vi "USB Get Device Info.vi"(10 "pFunctionStr":string, 11 "DevIndex":i32) -> (1 "function return":bool, 2 "pFunctionStr out":string, 3 "pDevInfo":T1)   [LabVIEW 2010, in "usb_device.lvlib"]
doc: "bool WINAPI USB_GetDeviceInfo(int DevIndex,PDEVICE_INFO pDevInfo,char *pFunctionStr);"
uses:
  usb_device.lvlib
  USB2XXX.dll
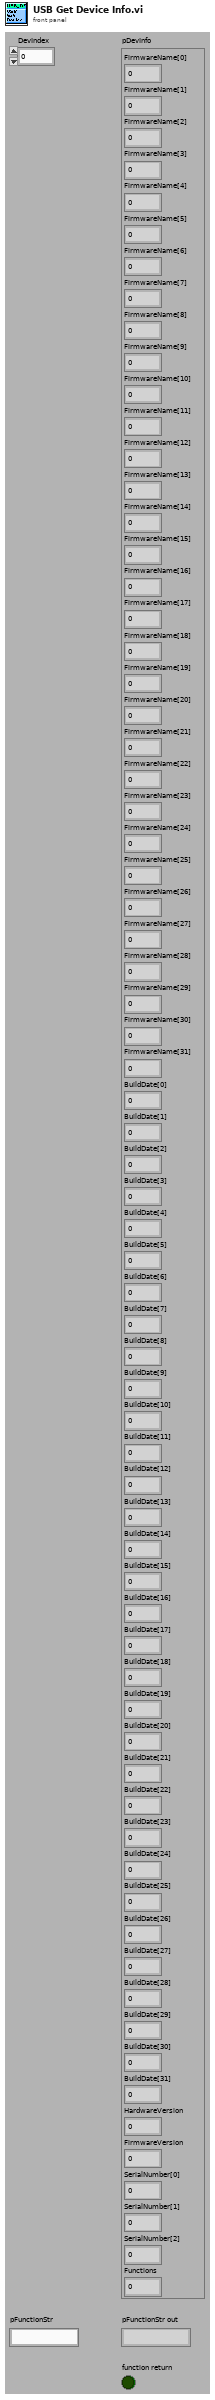
[diagram p1: front panel]
types:
  T1 = cluster{"FirmwareName[0]":i8, "FirmwareName[1]":i8, "FirmwareName[2]":i8, "FirmwareName[3]":i8, "FirmwareName[4]":i8, "FirmwareName[5]":i8, "FirmwareName[6]":i8, "FirmwareName[7]":i8, "FirmwareName[8]":i8, "FirmwareName[9]":i8, "FirmwareName[10]":i8, "FirmwareName[11]":i8, "FirmwareName[12]":i8, "FirmwareName[13]":i8, "FirmwareName[14]":i8, "FirmwareName[15]":i8, "FirmwareName[16]":i8, "FirmwareName[17]":i8, "FirmwareName[18]":i8, "FirmwareName[19]":i8, "FirmwareName[20]":i8, "FirmwareName[21]":i8, "FirmwareName[22]":i8, "FirmwareName[23]":i8, "FirmwareName[24]":i8, "FirmwareName[25]":i8, "FirmwareName[26]":i8, "FirmwareName[27]":i8, "FirmwareName[28]":i8, "FirmwareName[29]":i8, "FirmwareName[30]":i8, "FirmwareName[31]":i8, "BuildDate[0]":i8, "BuildDate[1]":i8, "BuildDate[2]":i8, "BuildDate[3]":i8, "BuildDate[4]":i8, "BuildDate[5]":i8, "BuildDate[6]":i8, "BuildDate[7]":i8, "BuildDate[8]":i8, "BuildDate[9]":i8, "BuildDate[10]":i8, "BuildDate[11]":i8, "BuildDate[12]":i8, "BuildDate[13]":i8, "BuildDate[14]":i8, "BuildDate[15]":i8, "BuildDate[16]":i8, "BuildDate[17]":i8, "BuildDate[18]":i8, "BuildDate[19]":i8, "BuildDate[20]":i8, "BuildDate[21]":i8, "BuildDate[22]":i8, "BuildDate[23]":i8, "BuildDate[24]":i8, "BuildDate[25]":i8, "BuildDate[26]":i8, "BuildDate[27]":i8, "BuildDate[28]":i8, "BuildDate[29]":i8, "BuildDate[30]":i8, "BuildDate[31]":i8, "HardwareVersion":i32, "FirmwareVersion":i32, "SerialNumber[0]":i32, "SerialNumber[1]":i32, "SerialNumber[2]":i32, "Functions":i32}
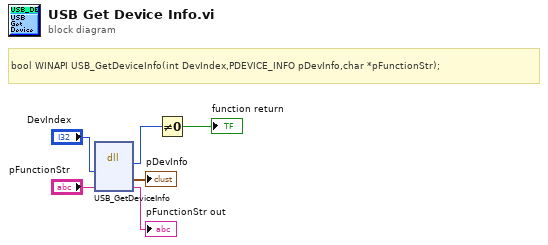
[diagram p0: block diagram]
diagram:
  # "bool WINAPI USB_GetDeviceInfo(int DevIndex,PDEVICE_INFO pDevInfo,char *pFunctionStr);"
  n1 = dll-call lib="G:/OtherWork/USB2XXX_Example/trunk/Labview/PublicFiles/usb_device/USB2XXX.*" fn="USB_GetDeviceInfo"("DevIndex"="DevIndex", "pFunctionStr"="pFunctionStr") -> (w5:u8, "pDevInfo"=→"pDevInfo":T1, "pFunctionStr"=→"pFunctionStr out":string)  [unwired: 5 in, 2 out]
  n2 = Not Equal To 0?(x=w5) -> (x != 0?=→"function return":bool)
